vi "File Move (incoming to Archive).vi"(0 "source location of files":path, 1 "Files to Archive and FTP IN":string[](array[string]), 5 "outgoing directory":path, 7 "redundant archive location":path, 9 "Archive 2 valid path":bool, 11 "error IO IN":errorcluster) -> (15 "Error OUT array":errorcluster[](array[cluster]))   [LabVIEW 2011]
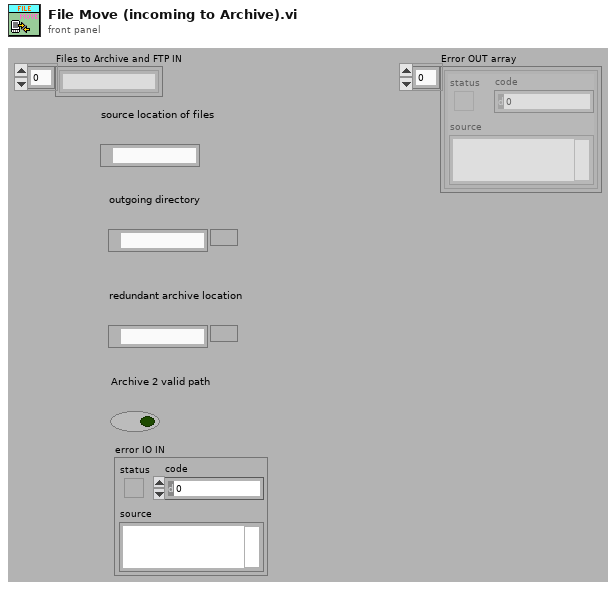
[diagram p1: front panel]
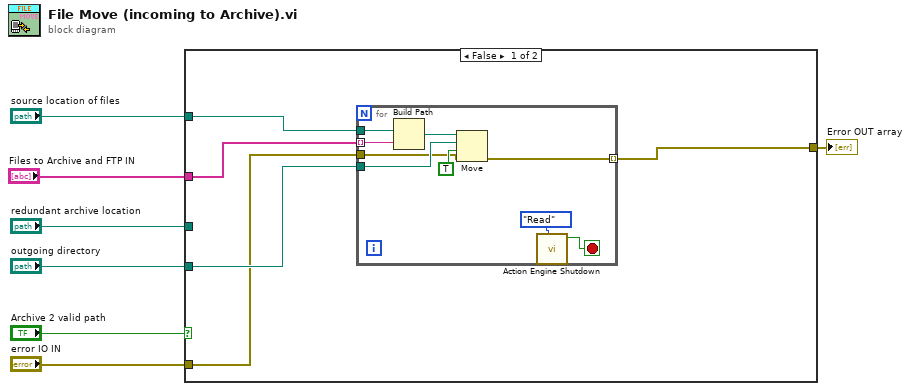
[diagram p0: block diagram]
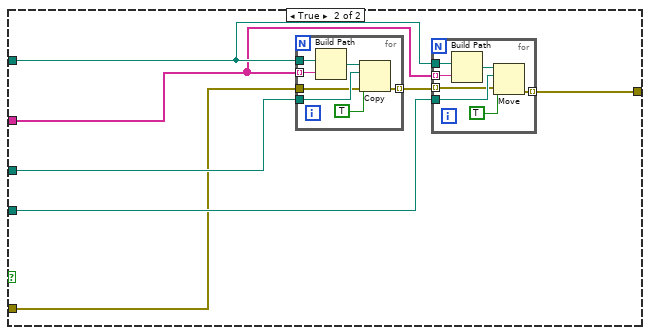
[diagram p2: hidden frame]
diagram:
  n1 = case shown="False" "Archive 2 valid path" {
    tunnel: "source location of files" -> [w11 w26]
    tunnel: "outgoing directory" -> [w12 w27]
    tunnel: "redundant archive location" -> [_ w28]
    tunnel: "error IO IN" -> [w10 w25]
    tunnel: [w9 w23] -> w2
    tunnel: "Files to Archive and FTP IN" -> [w8 w22]
    frame False {
      n2 = for {
        tunnel: w11 -> [w21]
        tunnel: w12 -> [w19]
        tunnel: w10 -> [w17]
        tunnel: [w16] -> w9 mode=indexing
        tunnel: w8 -> [w15] mode=indexing
        stop <- w13 stop-if-true
        n3 = Build Path(base path=w21, name or relative path=w15) -> (appended path=w20:path)
        n4 = Move(source path=w20, error in=w17, 9:TRUE ("overwrite (F)"), 10:w19) -> (error out=w16:errorcluster)  [unwired: 1 in, 2 out]
        n5 = call "Action Engine Shutdown.vi"("Shutdown"=enum16{"Write", "Read"}."Read") -> ("Shutdown"=w13:bool)  [unwired: 9 in, 1 out]
      }
    }
    frame True {
      n6 = for {
        tunnel: w26 -> [w35]
        tunnel: w28 -> [w33]
        tunnel: w25 -> [w31]
        tunnel: [w30] -> w24 mode=indexing
        tunnel: w22 -> [w29] mode=indexing
        n7 = Build Path(base path=w35, name or relative path=w29) -> (appended path=w34:path)
        n8 = Copy(8:w31, 9:TRUE ("overwrite (F)"), 10:w33, 11:w34) -> (0:w30:errorcluster)  [unwired: 1 in, 2 out]
      }
      n9 = for {
        tunnel: w26 -> [w42]
        tunnel: w27 -> [w40]
        tunnel: w24 -> [w38] mode=indexing
        tunnel: [w37] -> w23 mode=indexing
        tunnel: w22 -> [w36] mode=indexing
        n10 = Build Path(base path=w42, name or relative path=w36) -> (appended path=w41:path)
        n11 = Move(source path=w41, error in=w38, 9:TRUE ("overwrite (F)"), 10:w40) -> (error out=w37:errorcluster)  [unwired: 1 in, 2 out]
      }
    }
  }
  "Error OUT array" <- w2
